vi "Append Copyright to Description.vi"(9 "Copyright Text":string, 11 "Description":string) -> (3 "Description out":string)   [LabVIEW 2023, in "VI Properties Editor.lvlib"]
doc: "Appends <B>Copyright Text</B> to <B>Description</B>."
uses:
  VI Properties Editor.lvlib
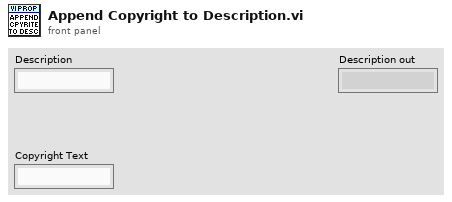
[diagram p1: front panel]
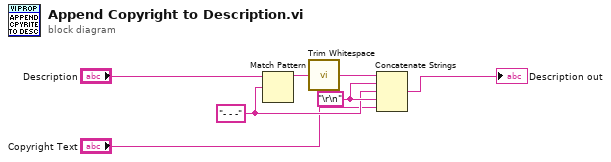
[diagram p0: block diagram]
diagram:
  w6 = "\r\n"
  w5 = "- - -"
  n1 = Match Pattern(string="Description", regular expression=w5) -> (before substring=w4:string)  [unwired: 1 in, 3 out]
  n2 = call <vilib>:"Trim Whitespace.vi"("string"=w4) -> ("trimmed string"=w7:string)  [unwired: 1 in]
  n3 = Concatenate Strings(w7, w6, w5, w6, "Copyright Text") -> (→"Description out":string)
